vi "cRIO Main VI.vi"() -> ()   [LabVIEW 2019]
uses:
  Initialize/Initialize.lvlib
  Acquire/Acquisition.lvlib
panel:
  out "Aquatrak Data Timestamp":timestamp
  out "Aquatrak Output":string
  out "error out":errorcluster
  out "T12":dbl(slide) scale=0.0..30.0
  out "T11":dbl(slide) scale=0.0..30.0
  out "T10":dbl(slide) scale=0.0..30.0
  out "T9":dbl(slide) scale=0.0..30.0
  out "T8":dbl(slide) scale=0.0..30.0
  out "T7":dbl(slide) scale=0.0..30.0
  out "T6":dbl(slide) scale=0.0..30.0
  out "T5":dbl(slide) scale=0.0..30.0
  out "T4":dbl(slide) scale=0.0..30.0
  out "T3":dbl(slide) scale=0.0..30.0
  out "T2":dbl(slide) scale=0.0..30.0
  out "T1":dbl(slide) scale=0.0..30.0
  out "Ring Time":waveform(dbl)[](graph)
  in  "Stop":bool
  in  "error in":errorcluster
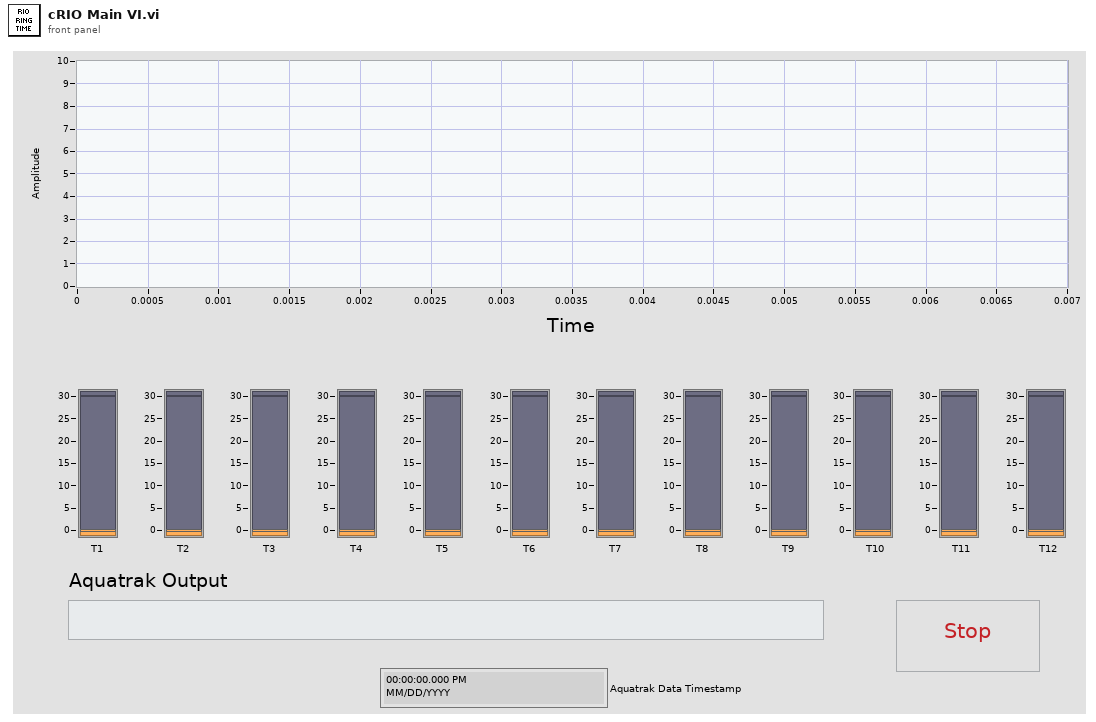
[diagram p1: front panel]
types:
  T1 = cluster{"Ring Time ADC Task":refnum<k21>, "Aquatrak COM Port":refnum<visa-resource-name>}
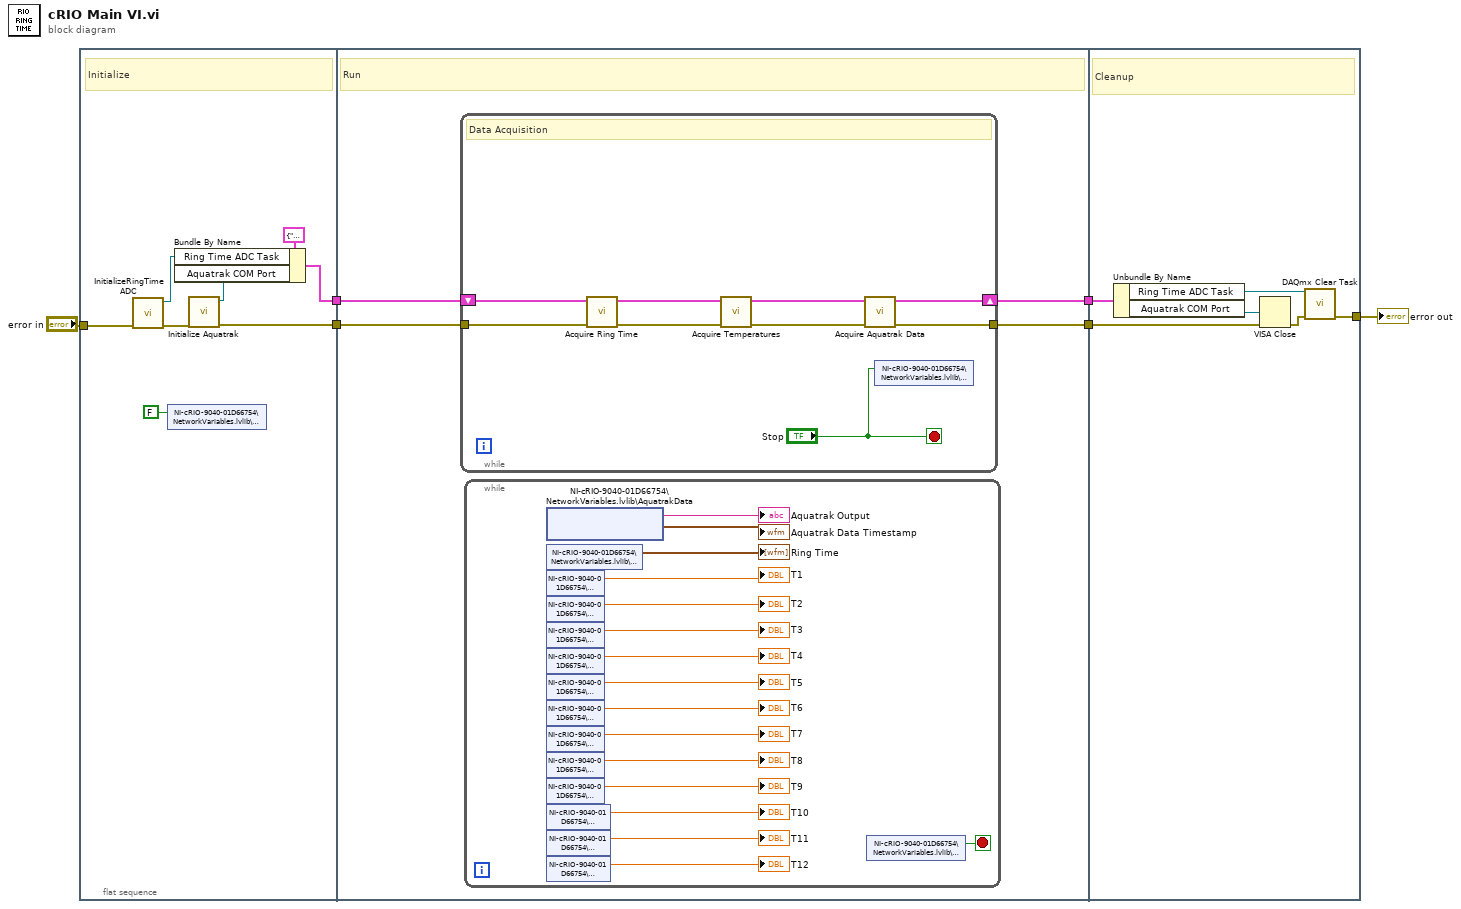
[diagram p0: block diagram]
diagram:
  n1 = flat-sequence {
    tunnel: "error in" -> [w14]
    tunnel: [w11] -> w5
    tunnel: [w8] -> w4
    tunnel: w5 -> [w18]
    tunnel: w4 -> [w17]
    tunnel: [w16] -> w3
    tunnel: [w15] -> w2
    tunnel: w3 -> [w49]
    tunnel: w2 -> [w46]
    tunnel: [w44] -> w1
    frame #0 {
      # "Initialize"
      n2 = call "InitializeRingTimeADC.vi"("error in (no error)"=w14) -> ("error out"=w10:errorcluster, "Ring Time ADC Task"=w13:refnum<k21>)  [unwired: 9 in]
      n3 = shared-variable "NI-cRIO-9040-01D66754\\NetworkVariables.lvlib\\STOPcRIO"(FALSE ("STOPcRIO")) -> ()  [unwired: 1 in, 1 out]
      n4 = call "Initialize Aquatrak.vi"("error in (no error)"=w10) -> ("error out"=w8:errorcluster, "Aquatrak COM Port"=w12:refnum<visa-resource-name>)  [unwired: 9 in]
      n5 = Bundle By Name(cluster=T1 {"Ring Time ADC Task"="", "Aquatrak COM Port"=""}, "Ring Time ADC Task"=w13, "Aquatrak COM Port"=w12) -> (w11:T1)
    }
    frame #1 {
      # "Run"
      n6 = while {
        tunnel: w17 -> [w26]
        shift-right: [w21] -> w16
        shift-left: w18 -> [w27]
        tunnel: [w20] -> w15
        stop <- "Stop" stop-if-true
        # "Data Acquisition"
        n7 = call "Acquire Ring Time.vi"("error in (no error)"=w26, "Settings In"=w27) -> ("error out"=w24:errorcluster, "Settings Out"=w25:T1)  [unwired: 8 in]
        n8 = call "Acquire Temperatures.vi"("Error In"=w24, "Settings in"=w25) -> ("Error Out"=w22:errorcluster, "Settings Out"=w23:T1)  [unwired: 8 in]
        n9 = call "Acquire Aquatrak Data.vi"("Error In"=w22, "Settings in"=w23) -> ("Error Out"=w20:errorcluster, "Settings out"=w21:T1)  [unwired: 7 in, 1 out]
        n10 = shared-variable "NI-cRIO-9040-01D66754\\NetworkVariables.lvlib\\STOPcRIO"("Stop") -> ()  [unwired: 1 in, 1 out]
      }
      n11 = while {
        stop <- w43 stop-if-true
        n12 = shared-variable "NI-cRIO-9040-01D66754\\NetworkVariables.lvlib\\AquatrakData"() -> (→"Aquatrak Output":string, →"Aquatrak Data Timestamp":timestamp)  [unwired: 1 in, 1 out]
        n13 = shared-variable "NI-cRIO-9040-01D66754\\NetworkVariables.lvlib\\RingTime"() -> (→"Ring Time":waveform(dbl)[])  [unwired: 1 in, 1 out]
        n14 = shared-variable "NI-cRIO-9040-01D66754\\NetworkVariables.lvlib\\T1"() -> (→"T1":dbl)  [unwired: 1 in, 1 out]
        n15 = shared-variable "NI-cRIO-9040-01D66754\\NetworkVariables.lvlib\\T2"() -> (→"T2":dbl)  [unwired: 1 in, 1 out]
        n16 = shared-variable "NI-cRIO-9040-01D66754\\NetworkVariables.lvlib\\T3"() -> (→"T3":dbl)  [unwired: 1 in, 1 out]
        n17 = shared-variable "NI-cRIO-9040-01D66754\\NetworkVariables.lvlib\\T4"() -> (→"T4":dbl)  [unwired: 1 in, 1 out]
        n18 = shared-variable "NI-cRIO-9040-01D66754\\NetworkVariables.lvlib\\T5"() -> (→"T5":dbl)  [unwired: 1 in, 1 out]
        n19 = shared-variable "NI-cRIO-9040-01D66754\\NetworkVariables.lvlib\\T6"() -> (→"T6":dbl)  [unwired: 1 in, 1 out]
        n20 = shared-variable "NI-cRIO-9040-01D66754\\NetworkVariables.lvlib\\T7"() -> (→"T7":dbl)  [unwired: 1 in, 1 out]
        n21 = shared-variable "NI-cRIO-9040-01D66754\\NetworkVariables.lvlib\\T8"() -> (→"T8":dbl)  [unwired: 1 in, 1 out]
        n22 = shared-variable "NI-cRIO-9040-01D66754\\NetworkVariables.lvlib\\T9"() -> (→"T9":dbl)  [unwired: 1 in, 1 out]
        n23 = shared-variable "NI-cRIO-9040-01D66754\\NetworkVariables.lvlib\\T10"() -> (→"T10":dbl)  [unwired: 1 in, 1 out]
        n24 = shared-variable "NI-cRIO-9040-01D66754\\NetworkVariables.lvlib\\T11"() -> (→"T11":dbl)  [unwired: 1 in, 1 out]
        n25 = shared-variable "NI-cRIO-9040-01D66754\\NetworkVariables.lvlib\\T12"() -> (→"T12":dbl)  [unwired: 1 in, 1 out]
        n26 = shared-variable "NI-cRIO-9040-01D66754\\NetworkVariables.lvlib\\STOPcRIO"() -> (w43:bool)  [unwired: 1 in, 1 out]
      }
    }
    frame #2 {
      # "Cleanup"
      n27 = Unbundle By Name(w49) -> ("Ring Time ADC Task"=w48:refnum<k21>, "Aquatrak COM Port"=w47:refnum<visa-resource-name>)
      n28 = VISA Close(VISA resource name=w47, error in (no error)=w46) -> (error out=w45:errorcluster)
      n29 = call <vilib>:"DAQmx Clear Task.vi"("task in"=w48, "error in"=w45) -> ("error out"=w44:errorcluster)  [unwired: 13 in]
    }
  }
  "error out" <- w1
